vi "SENO.vi"() -> ()   [LabVIEW 2020]
panel:
  out "Waveform Chart":dbl(graph)
  in  "?":bool
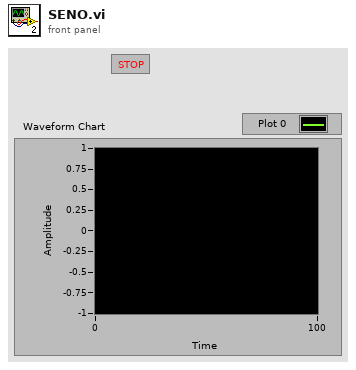
[diagram p1: front panel]
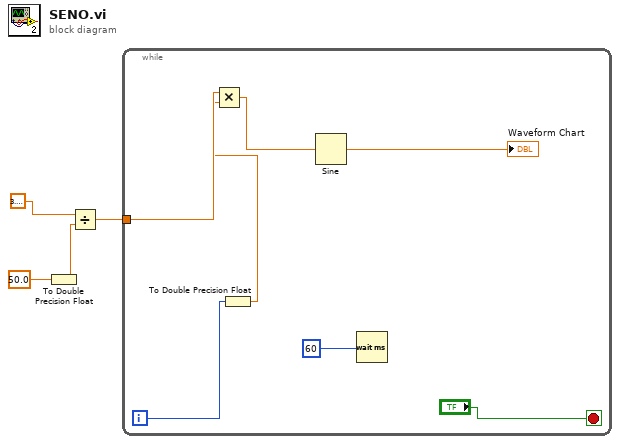
[diagram p0: block diagram]
diagram:
  n1 = To Double Precision Float(number=50.0) -> (double precision float=w2:dbl)
  n2 = Divide(x=3.141592653589793, y=w2) -> (x/y=w1:dbl)
  n3 = while {
    tunnel: w1 -> [w11]
    i -> [w10]
    stop <- "?" stop-if-true
    n4 = To Double Precision Float(number=w10) -> (double precision float=w9:dbl)
    n5 = Multiply(x=w11, y=w9) -> (x*y=w7:dbl)
    n6 = Sine(x=w7) -> (sin(x)=→"Waveform Chart":dbl)
    n7 = Wait (ms)(milliseconds to wait=60) -> ()  [unwired: 1 out]
  }
